vi "VI Tree.vi"   [LabVIEW 2009, in "Keithley 2600 Series.lvlib"]
doc: "This is the instrument driver for the KE26xx. The VI Tree displays all the user-callable VIs of the instrument driver in an organized table."
uses:
  <instrlib>/Keithley 2600 Series/Keithley 2600 Series.lvlib
panel:
  # "(c) 2007-2008 Keithley Instruments, Inc.  ALL RIGHTS RESERVED."
  # "SEE DIAGRAM\nFOR VI TREE."
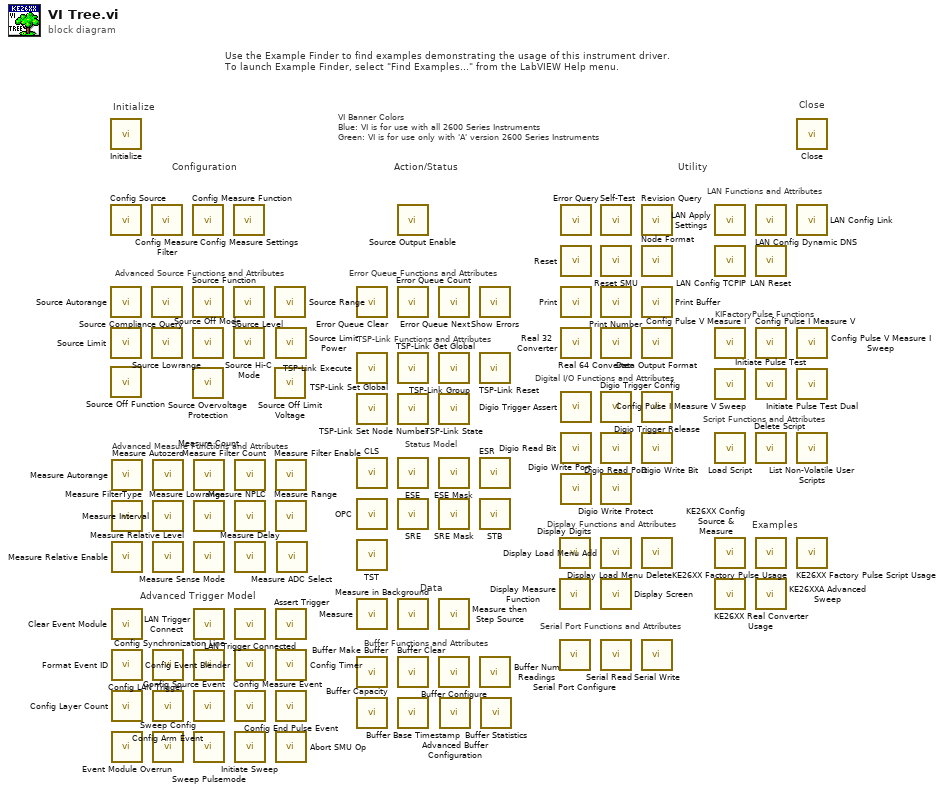
[diagram p0: block diagram]
diagram:
  # "VI Banner Colors\nBlue: VI is for use with all 2600 Series Instruments\nGreen: VI is for use only with 'A' version 2600 Series Instruments"
  # "Examples"
  # "Script Functions and Attributes"
  # "KIFactoryPulse Functions"
  # "LAN Functions and Attributes"
  # "Serial Port Functions and Attributes"
  # "Display Functions and Attributes"
  # "Digital I/O Functions and Attributes"
  # "Buffer Functions and Attributes"
  # "Status Model"
  # "TSP-Link Functions and Attributes"
  # "Error Queue Functions and Attributes"
  # "Advanced Trigger Model"
  # "Advanced Measure Functions and Attributes"
  # "Advanced Source Functions and Attributes"
  # "Use the Example Finder to find examples demonstrating the usage of this instrument driver.\nTo launch Example Finder, select \"Find Examples...\" from the LabVIEW Help menu."
  # "Configuration"
  # "Utility"
  # "Data"
  # "Action/Status"
  # "Close"
  # "Initialize"
  n1 = call <instrlib>:"Initialize.vi"() -> ()  [unwired: 10 in, 2 out]
  n2 = call <instrlib>:"Config Source.vi"() -> ()  [unwired: 12 in, 4 out]
  n3 = call <instrlib>:"Source Autorange.vi"() -> ()  [unwired: 8 in, 4 out]
  n4 = call <instrlib>:"Source Limit.vi"() -> ()  [unwired: 8 in, 4 out]
  n5 = call <instrlib>:"Source Off Function.vi"() -> ()  [unwired: 8 in, 4 out]
  n6 = call <instrlib>:"Measure Autorange.vi"() -> ()  [unwired: 8 in, 4 out]
  n7 = call <instrlib>:"Measure FilterType.vi"() -> ()  [unwired: 8 in, 4 out]
  n8 = call <instrlib>:"Measure Relative Enable.vi"() -> ()  [unwired: 8 in, 4 out]
  n9 = call <instrlib>:"Clear Event Module.vi"() -> ()  [unwired: 8 in, 4 out]
  n10 = call <instrlib>:"Format Event ID.vi"() -> ()  [unwired: 10 in, 2 out]
  n11 = call <instrlib>:"Config Layer Count.vi"() -> ()  [unwired: 8 in, 4 out]
  n12 = call <instrlib>:"Event Module Overrun.vi"() -> ()  [unwired: 7 in, 5 out]
  n13 = call <instrlib>:"Config Measure Filter.vi"() -> ()  [unwired: 8 in, 4 out]
  n14 = call <instrlib>:"Source Compliance Query.vi"() -> ()  [unwired: 7 in, 5 out]
  n15 = call <instrlib>:"Source Lowrange.vi"() -> ()  [unwired: 8 in, 4 out]
  n16 = call <instrlib>:"Measure Autozero.vi"() -> ()  [unwired: 8 in, 4 out]
  n17 = call <instrlib>:"Measure Interval.vi"() -> ()  [unwired: 8 in, 4 out]
  n18 = call <instrlib>:"Measure Relative Level.vi"() -> ()  [unwired: 8 in, 4 out]
  n19 = call <instrlib>:"Config LAN Trigger.vi"() -> ()  [unwired: 12 in, 4 out]
  n20 = call <instrlib>:"Config Arm Event.vi"() -> ()  [unwired: 8 in, 4 out]
  n21 = call <instrlib>:"Sweep Config.vi"() -> ()  [unwired: 12 in, 4 out]
  n22 = call <instrlib>:"Config Measure Function.vi"() -> ()  [unwired: 12 in, 4 out]
  n23 = call <instrlib>:"Source Function.vi"() -> ()  [unwired: 8 in, 4 out]
  n24 = call <instrlib>:"Source Off Mode.vi"() -> ()  [unwired: 8 in, 4 out]
  n25 = call <instrlib>:"Source Overvoltage Protection.vi"() -> ()  [unwired: 13 in, 3 out]
  n26 = call <instrlib>:"Measure Count.vi"() -> ()  [unwired: 8 in, 4 out]
  n27 = call <instrlib>:"Measure Lowrange.vi"() -> ()  [unwired: 8 in, 4 out]
  n28 = call <instrlib>:"Measure Sense Mode.vi"() -> ()  [unwired: 8 in, 4 out]
  n29 = call <instrlib>:"LAN Trigger Connect.vi"() -> ()  [unwired: 8 in, 4 out]
  n30 = call <instrlib>:"Config Synchronization Line.vi"() -> ()  [unwired: 8 in, 4 out]
  n31 = call <instrlib>:"Config Source Event.vi"() -> ()  [unwired: 8 in, 4 out]
  n32 = call <instrlib>:"Sweep Pulsemode.vi"() -> ()  [unwired: 8 in, 4 out]
  n33 = call <instrlib>:"Config Measure Settings.vi"() -> ()  [unwired: 12 in, 4 out]
  n34 = call <instrlib>:"Source Level.vi"() -> ()  [unwired: 8 in, 4 out]
  n35 = call <instrlib>:"Source Hi-C Mode.vi"() -> ()  [unwired: 12 in, 4 out]
  n36 = call <instrlib>:"Measure Filter Count.vi"() -> ()  [unwired: 8 in, 4 out]
  n37 = call <instrlib>:"Measure NPLC.vi"() -> ()  [unwired: 8 in, 4 out]
  n38 = call <instrlib>:"Measure Delay.vi"() -> ()  [unwired: 8 in, 4 out]
  n39 = call <instrlib>:"LAN Trigger Connected.vi"() -> ()  [unwired: 7 in, 5 out]
  n40 = call <instrlib>:"Config Event Blender.vi"() -> ()  [unwired: 12 in, 4 out]
  n41 = call <instrlib>:"Config Measure Event.vi"() -> ()  [unwired: 12 in, 4 out]
  n42 = call <instrlib>:"Initiate Sweep.vi"() -> ()  [unwired: 8 in, 4 out]
  n43 = call <instrlib>:"Source Range.vi"() -> ()  [unwired: 8 in, 4 out]
  n44 = call <instrlib>:"Source Off Limit Voltage.vi"() -> ()  [unwired: 8 in, 4 out]
  n45 = call <instrlib>:"Source Limit Power.vi"() -> ()  [unwired: 13 in, 3 out]
  n46 = call <instrlib>:"Measure Filter Enable.vi"() -> ()  [unwired: 8 in, 4 out]
  n47 = call <instrlib>:"Measure Range.vi"() -> ()  [unwired: 8 in, 4 out]
  n48 = call <instrlib>:"Assert Trigger.vi"() -> ()  [unwired: 8 in, 4 out]
  n49 = call <instrlib>:"Config Timer.vi"() -> ()  [unwired: 12 in, 4 out]
  n50 = call <instrlib>:"Config End Pulse Event.vi"() -> ()  [unwired: 8 in, 4 out]
  n51 = call <instrlib>:"Abort SMU Op.vi"() -> ()  [unwired: 8 in, 4 out]
  n52 = call <instrlib>:"Measure ADC Select.vi"() -> ()  [unwired: 13 in, 3 out]
  n53 = call <instrlib>:"Error Queue Clear.vi"() -> ()  [unwired: 8 in, 4 out]
  n54 = call <instrlib>:"TSP-Link Execute.vi"() -> ()  [unwired: 8 in, 4 out]
  n55 = call <instrlib>:"TSP-Link Set Global.vi"() -> ()  [unwired: 9 in, 3 out]
  n56 = call <instrlib>:"CLS.vi"() -> ()  [unwired: 8 in, 4 out]
  n57 = call <instrlib>:"OPC.vi"() -> ()  [unwired: 9 in, 3 out]
  n58 = call <instrlib>:"TST.vi"() -> ()  [unwired: 8 in, 4 out]
  n59 = call <instrlib>:"Measure.vi"() -> ()  [unwired: 7 in, 5 out]
  n60 = call <instrlib>:"Buffer Make Buffer.vi"() -> ()  [unwired: 8 in, 4 out]
  n61 = call <instrlib>:"Buffer Capacity.vi"() -> ()  [unwired: 8 in, 4 out]
  n62 = call <instrlib>:"Source Output Enable.vi"() -> ()  [unwired: 8 in, 4 out]
  n63 = call <instrlib>:"Error Queue Count.vi"() -> ()  [unwired: 7 in, 5 out]
  n64 = call <instrlib>:"TSP-Link Get Global.vi"() -> ()  [unwired: 8 in, 4 out]
  n65 = call <instrlib>:"TSP-Link Set Node Number.vi"() -> ()  [unwired: 9 in, 3 out]
  n66 = call <instrlib>:"ESE.vi"() -> ()  [unwired: 7 in, 5 out]
  n67 = call <instrlib>:"SRE.vi"() -> ()  [unwired: 7 in, 5 out]
  n68 = call <instrlib>:"Measure in Background.vi"() -> ()  [unwired: 8 in, 4 out]
  n69 = call <instrlib>:"Buffer Clear.vi"() -> ()  [unwired: 9 in, 3 out]
  n70 = call <instrlib>:"Buffer Base Timestamp.vi"() -> ()  [unwired: 8 in, 4 out]
  n71 = call <instrlib>:"Error Queue Next.vi"() -> ()  [unwired: 7 in, 5 out]
  n72 = call <instrlib>:"TSP-Link Group.vi"() -> ()  [unwired: 8 in, 4 out]
  n73 = call <instrlib>:"TSP-Link State.vi"() -> ()  [unwired: 8 in, 4 out]
  n74 = call <instrlib>:"ESE Mask.vi"() -> ()  [unwired: 8 in, 4 out]
  n75 = call <instrlib>:"SRE Mask.vi"() -> ()  [unwired: 8 in, 4 out]
  n76 = call <instrlib>:"Measure then Step Source.vi"() -> ()  [unwired: 7 in, 5 out]
  n77 = call <instrlib>:"Buffer Configure.vi"() -> ()  [unwired: 9 in, 3 out]
  n78 = call <instrlib>:"Advanced Buffer Configuration.vi"() -> ()  [unwired: 14 in, 2 out]
  n79 = call <instrlib>:"Show Errors.vi"() -> ()  [unwired: 8 in, 4 out]
  n80 = call <instrlib>:"TSP-Link Reset.vi"() -> ()  [unwired: 9 in, 3 out]
  n81 = call <instrlib>:"ESR.vi"() -> ()  [unwired: 7 in, 5 out]
  n82 = call <instrlib>:"STB.vi"() -> ()  [unwired: 7 in, 5 out]
  n83 = call <instrlib>:"Buffer Num Readings.vi"() -> ()  [unwired: 8 in, 4 out]
  n84 = call <instrlib>:"Buffer Statistics.vi"() -> ()  [unwired: 12 in, 4 out]
  n85 = call <instrlib>:"Display Digits.vi"() -> ()  [unwired: 8 in, 4 out]
  n86 = call <instrlib>:"Display Measure Function.vi"() -> ()  [unwired: 8 in, 4 out]
  n87 = call <instrlib>:"Serial Port Configure.vi"() -> ()  [unwired: 8 in, 4 out]
  n88 = call <instrlib>:"Error Query.vi"() -> ()  [unwired: 8 in, 4 out]
  n89 = call <instrlib>:"Reset.vi"() -> ()  [unwired: 10 in, 2 out]
  n90 = call <instrlib>:"Print.vi"() -> ()  [unwired: 7 in, 5 out]
  n91 = call <instrlib>:"Real 32 Converter.vi"() -> ()  [unwired: 11 in, 1 out]
  n92 = call <instrlib>:"Digio Trigger Assert.vi"() -> ()  [unwired: 8 in, 4 out]
  n93 = call <instrlib>:"Digio Read Bit.vi"() -> ()  [unwired: 7 in, 5 out]
  n94 = call <instrlib>:"Digio Write Port.vi"() -> ()  [unwired: 8 in, 4 out]
  n95 = call <instrlib>:"Self-Test.vi"() -> ()  [unwired: 8 in, 4 out]
  n96 = call <instrlib>:"Reset SMU.vi"() -> ()  [unwired: 8 in, 4 out]
  n97 = call <instrlib>:"Print Number.vi"() -> ()  [unwired: 8 in, 4 out]
  n98 = call <instrlib>:"Real 64 Converter.vi"() -> ()  [unwired: 11 in, 1 out]
  n99 = call <instrlib>:"Digio Trigger Config.vi"() -> ()  [unwired: 8 in, 4 out]
  n100 = call <instrlib>:"Digio Read Port.vi"() -> ()  [unwired: 7 in, 5 out]
  n101 = call <instrlib>:"Digio Write Protect.vi"() -> ()  [unwired: 8 in, 4 out]
  n102 = call <instrlib>:"Display Load Menu Add.vi"() -> ()  [unwired: 8 in, 4 out]
  n103 = call <instrlib>:"Display Screen.vi"() -> ()  [unwired: 8 in, 4 out]
  n104 = call <instrlib>:"Serial Read.vi"() -> ()  [unwired: 7 in, 5 out]
  n105 = call <instrlib>:"Revision Query.vi"() -> ()  [unwired: 8 in, 4 out]
  n106 = call <instrlib>:"Node Format.vi"() -> ()  [unwired: 10 in, 2 out]
  n107 = call <instrlib>:"Print Buffer.vi"() -> ()  [unwired: 11 in, 5 out]
  n108 = call <instrlib>:"Data Output Format.vi"() -> ()  [unwired: 8 in, 4 out]
  n109 = call <instrlib>:"Digio Trigger Release.vi"() -> ()  [unwired: 8 in, 4 out]
  n110 = call <instrlib>:"Digio Write Bit.vi"() -> ()  [unwired: 8 in, 4 out]
  n111 = call <instrlib>:"Display Load Menu Delete.vi"() -> ()  [unwired: 8 in, 4 out]
  n112 = call <instrlib>:"Serial Write.vi"() -> ()  [unwired: 8 in, 4 out]
  n113 = call <instrlib>:"LAN Apply Settings.vi"() -> ()  [unwired: 8 in, 4 out]
  n114 = call <instrlib>:"LAN Config TCPIP.vi"() -> ()  [unwired: 12 in, 4 out]
  n115 = call <instrlib>:"Config Pulse V Measure I.vi"() -> ()  [unwired: 15 in, 5 out]
  n116 = call <instrlib>:"Config Pulse I Measure V Sweep.vi"() -> ()  [unwired: 23 in, 5 out]
  n117 = call <instrlib>:"Load Script.vi"() -> ()  [unwired: 9 in, 3 out]
  n118 = call <instrlib>:"KE26XX Config Source & Measure.vi"() -> ()  [unwired: 10 in, 2 out]
  n119 = call <instrlib>:"KE26XX Real Converter Usage.vi"() -> ()  [unwired: 10 in, 2 out]
  n120 = call <instrlib>:"LAN Config Dynamic DNS.vi"() -> ()  [unwired: 12 in, 4 out]
  n121 = call <instrlib>:"LAN Reset.vi"() -> ()  [unwired: 8 in, 4 out]
  n122 = call <instrlib>:"Config Pulse I Measure V.vi"() -> ()  [unwired: 15 in, 5 out]
  n123 = call <instrlib>:"Initiate Pulse Test.vi"() -> ()  [unwired: 7 in, 5 out]
  n124 = call <instrlib>:"Delete Script.vi"() -> ()  [unwired: 9 in, 3 out]
  n125 = call <instrlib>:"KE26XX Factory Pulse Usage.vi"() -> ()  [unwired: 16 in, 4 out]
  n126 = call <instrlib>:"KE26XXA Advanced Sweep.vi"() -> ()  [unwired: 18 in, 2 out]
  n127 = call <instrlib>:"Close.vi"() -> ()  [unwired: 11 in, 1 out]
  n128 = call <instrlib>:"LAN Config Link.vi"() -> ()  [unwired: 12 in, 4 out]
  n129 = call <instrlib>:"Config Pulse V Measure I Sweep.vi"() -> ()  [unwired: 23 in, 5 out]
  n130 = call <instrlib>:"Initiate Pulse Test Dual.vi"() -> ()  [unwired: 7 in, 5 out]
  n131 = call <instrlib>:"List Non-Volatile User Scripts.vi"() -> ()  [unwired: 8 in, 4 out]
  n132 = call <instrlib>:"KE26XX Factory Pulse Script Usage.vi"() -> ()  [unwired: 10 in, 2 out]
